vi "PicoScope4000SetRapidSegments.vi"(5 "RapidBlock":bool, 7 "nSegments":T1 format="%.4p", 8 "error in (no error)":errorcluster, 11 "handle in":i16) -> (0 "error out":errorcluster, 3 "handle out":i16, 6 "nCaptures":u64)   [LabVIEW 2009]
doc: "Calls ps5000aMemorySegments, and ps5000aSetNoOfCaptures"
uses:
  ps4000.dll
  shared/nSegments.ctl
panel:
  out "nMaxSamples":u64
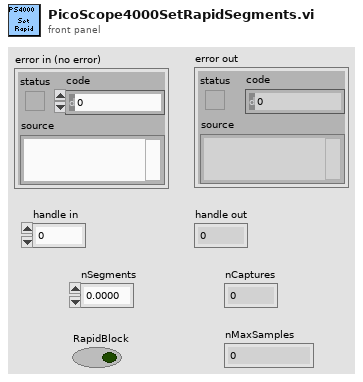
[diagram p1: front panel]
types:
  T1 = typedef "nSegments.ctl" = u64
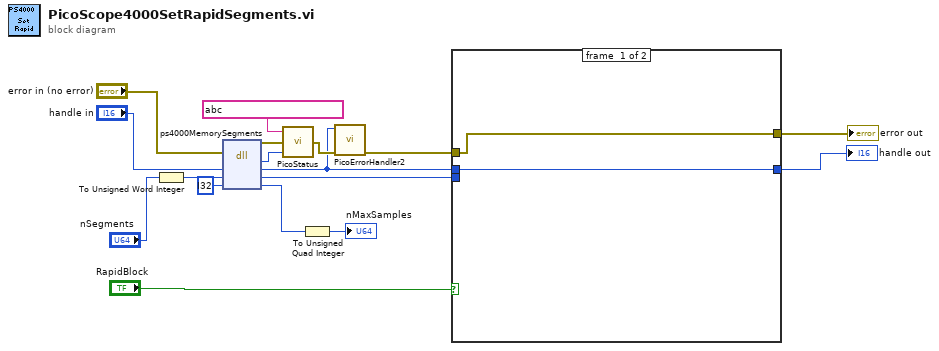
[diagram p0: block diagram]
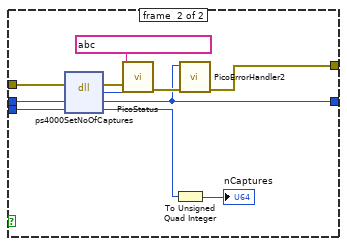
[diagram p2: hidden frame]
diagram:
  n1 = To Unsigned Word Integer(number="nSegments") -> (unsigned 16bit integer=w2:u16)
  n2 = dll-call lib="ps4000.dll" fn="ps4000MemorySegments" ("ps3000.dll:_ps3000_open_unit@0")(error in="error in (no error)", "handle"="handle in", "nSegments"=w2, "nMaxSamples"=i32 ?) -> (error out=w16:errorcluster, "PICO_STATUS"=w17:u32, "handle"=w12:i16, "nSegments"=w14:u16, "nMaxSamples"=w4:i32)  [unwired: 2 in, 1 out]
  n3 = call "PicoStatus.vi"("PICO STATUS"=w17, "error in"=w16, "source"=string ?) -> ("error out"=w13:errorcluster)
  n4 = To Unsigned Quad Integer(1:w4) -> (0:→"nMaxSamples":u64)
  n5 = call "PicoErrorHandler2.vi"("error in (no error)"=w13, "handle In"=w12) -> ("error out"=w11:errorcluster)  [unwired: 9 in]
  n6 = case shown="True" "RapidBlock" {
    tunnel: w14 -> [_ w30]
    tunnel: w12 -> [w18 w27]
    tunnel: w11 -> [w19 w24]
    tunnel: [w19 w23] -> w8
    tunnel: [w18 w22] -> w7
    frame #0 {
    }
    frame #1 {
      n7 = dll-call lib="ps4000.dll" fn="ps4000SetNoOfCaptures" ("ps3000.dll:_ps3000_open_unit@0")(error in=w24, "handle"=w27, "nCaptures"=w30) -> (error out=w29:errorcluster, "PICO_STATUS"=w25:u32, "handle"=w22:i16, "nCaptures"=w20:u16)  [unwired: 2 in, 1 out]
      n8 = call "PicoStatus.vi"("PICO STATUS"=w25, "error in"=w29, "source"=string ?) -> ("error out"=w26:errorcluster)
      n9 = To Unsigned Quad Integer(1:w20) -> (0:→"nCaptures":u64)
      n10 = call "PicoErrorHandler2.vi"("error in (no error)"=w26, "handle In"=w22) -> ("error out"=w23:errorcluster)  [unwired: 9 in]
    }
  }
  "error out" <- w8
  "handle out" <- w7
